vi "Initialize.vi"(8 "error in (no error)":errorcluster, 11 "Device in":refnum<class "MB_TCP_Device.lvclass">) -> (0 "error out":errorcluster, 3 "Device out":refnum<class "MB_TCP_Device.lvclass">)   [LabVIEW 2023, in "MB_TCP_Device.lvclass"]
uses:
  MB_TCP_Device.lvclass
  D:/SamparkProdLine/subVIs/DAQ Device/Modbus_Device/DAQ_Device.lvclass
  MB_TCP_Device.lvclass/MB_TCP_Device.ctl
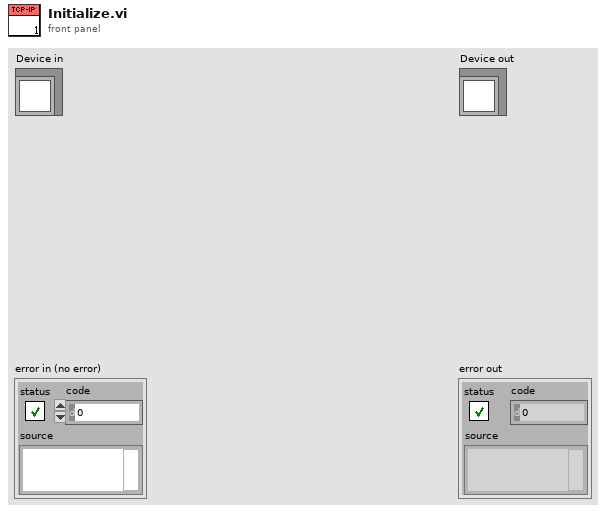
[diagram p1: front panel]
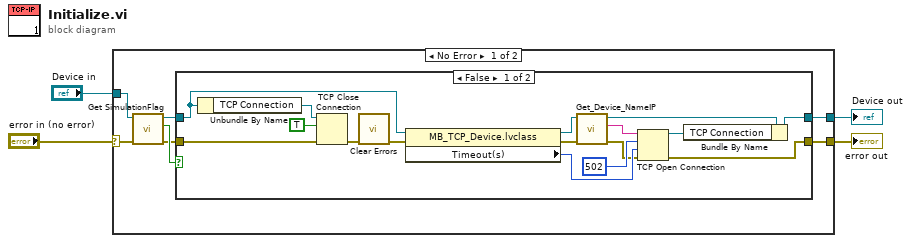
[diagram p0: block diagram]
diagram:
  n1 = case shown="No Error" "error in (no error)" {
    selector: "error in (no error)" -> [w6 w31]
    tunnel: [w10 w31] -> w3
    tunnel: [w11 w30] -> w1
    tunnel: "Device in" -> [w8 w30]
    frame No Error {
      n2 = call-dynamic "Get SimulationFlag.vi"("error in (no error)"=w6, "Device in"=w8) -> ("error out"=w5:errorcluster, "Simulation?"=w7:bool, "Device out"=w9:refnum<class "MB_TCP_Device.lvclass">)  [unwired: 7 in]
      n3 = case shown="False" w7 {
        tunnel: w9 -> [w17 w29]
        tunnel: [w27 w29] -> w11
        tunnel: [w26 w28] -> w10
        tunnel: w5 -> [w22 w28]
        frame False {
          n4 = Unbundle By Name(w17) -> ("TCP Connection"=w24:refnum<k5>)
          n5 = TCP Close Connection(connection ID=w24, abort (F)=TRUE, error in (no error)=w22) -> (error out=w23:errorcluster)  [unwired: 1 out]
          n6 = call <vilib>:"Clear Errors.vi"("error in (no error)"=w23) -> ("error out"=w15:errorcluster)  [unwired: 5 in, 1 out]
          n7 = property class="MB_TCP_Device.lvclass"(reference=w17, error in=w15) -> (reference out=w16:refnum<class "MB_TCP_Device.lvclass">, error out=w14:errorcluster, "Timeout(s)"=w13:i32)
          n8 = call-dynamic "Get_Device_NameIP.vi"("error in (no error)"=w14, "Device in"=w16) -> ("error out"=w12:errorcluster, "Device Address"=w19:string, "Device out"=w20:refnum<class "MB_TCP_Device.lvclass">)  [unwired: 4 in, 3 out]
          n9 = TCP Open Connection(address=w19, remote port or service name=u16 502, timeout ms (60000)=w13, error in (no error)=w12) -> (connection ID=w25:refnum<k5>, error out=w26:errorcluster)  [unwired: 1 in]
          n10 = Bundle By Name(cluster=w20, "TCP Connection"=w25) -> (w27:refnum<class "MB_TCP_Device.lvclass">)
        }
        frame True {
        }
      }
    }
    frame Error {
    }
  }
  "error out" <- w3
  "Device out" <- w1
